vi "Тест_буфера_без_вырезания.vi"() -> ()   [LabVIEW 2017]
panel:
  out "2-х массив на выходе 2":dbl[][](array[numeric])
  out "Кол-во строк массив":i32
  in  "Размер окна":i32=4
  out "Выход последовательного массива":dbl[](array[numeric])
  in  "Последовательный массив":i32=16
  out "Array":dbl[][](array[numeric])
  in  "Размер окна буффера":i32
  out "Количество бит":i32
  in  "Количество бит":i32=8
  out "Биты на выходе":dbl[](array[numeric])
  # "3"
  # "15"
  # "7"
  # "3"
  # "7"
  # "15"
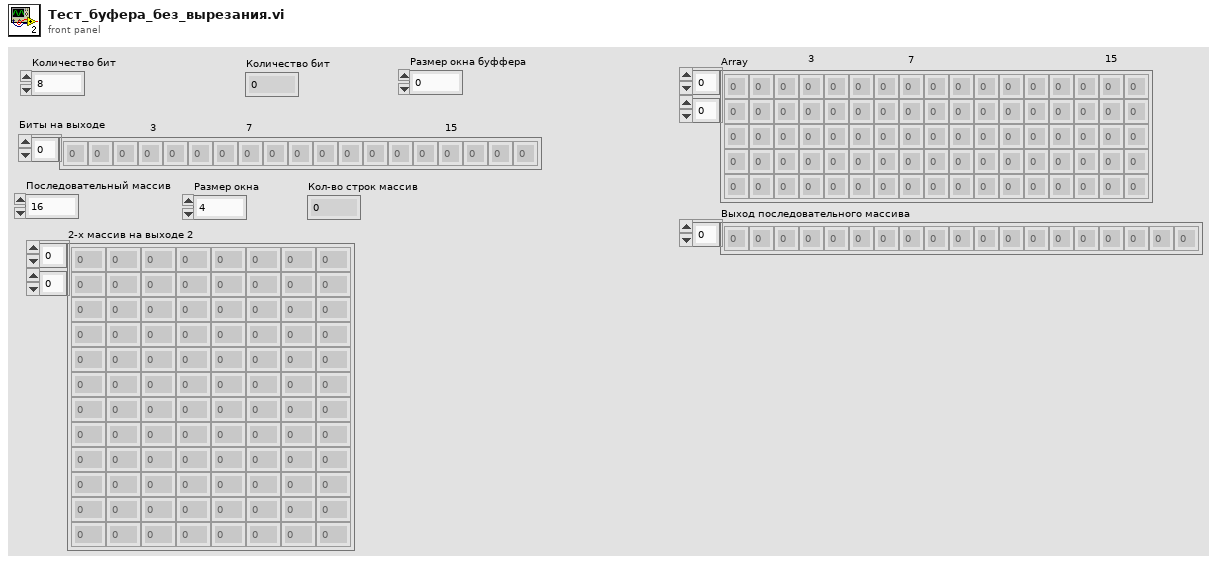
[diagram p1: front panel]
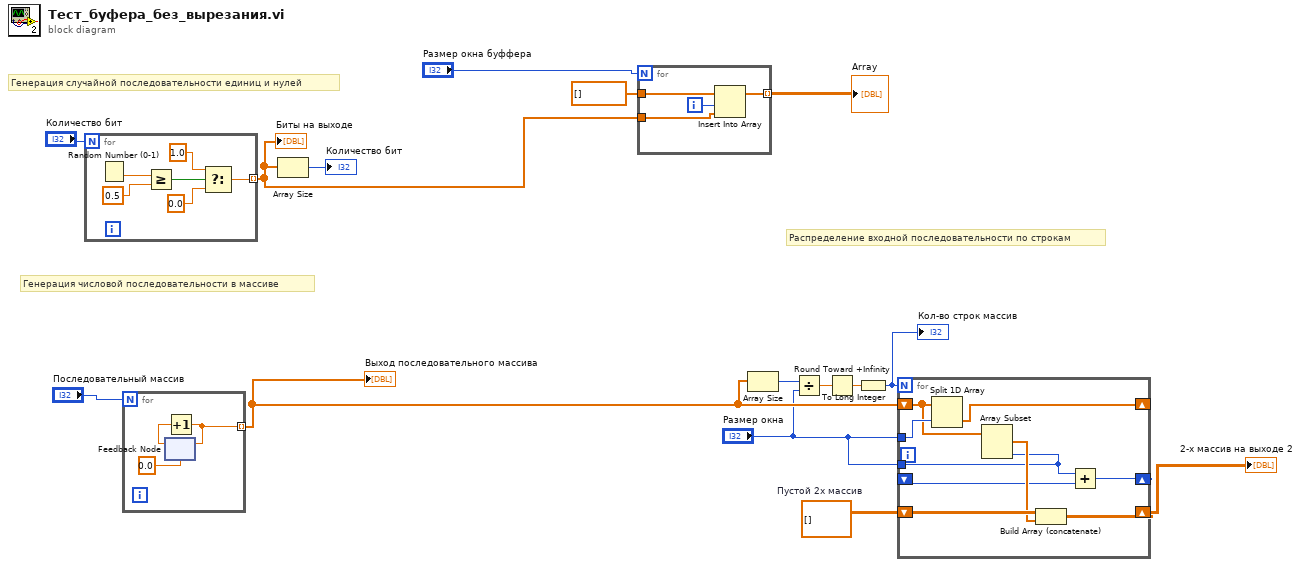
[diagram p0: block diagram]
diagram:
  w3 = dbl[][] []  # Пустой 2х массив
  # "Распределение входной последовательности по строкам"
  # "Генерация числовой последовательности в массиве"
  # "Генерация случайной последовательности единиц и нулей"
  n1 = for {
    N: "Количество бит" -> [_]
    tunnel: [w16] -> w10 mode=indexing
    n2 = Random Number (0-1)() -> (number: 0 to 1=w21:dbl)
    n3 = Greater Or Equal?(x=w21, y=0.5) -> (x >= y?=w19:bool)
    n4 = Select(t=1.0, s=w19, f=0.0) -> (s? t:f=w16:dbl)
  }
  "Биты на выходе" <- w10
  n5 = for {
    N: "Последовательный массив" -> [_]
    tunnel: [w22] -> w7 mode=indexing
    n6 = feedback #1(0.0) -> (w24:dbl)
    n7 = Increment(x=w24) -> (x+1=w22:dbl)
    n8 = feedback-in #1(w22) -> ()
  }
  "Выход последовательного массива" <- w7
  n9 = Array Size(array=w10) -> (size(s)=→"Количество бит":i32)
  n10 = for {
    N: "Размер окна буффера" -> [_]
    tunnel: w10 -> [w26]
    tunnel: dbl[] [] -> [w27]
    tunnel: [w28] -> w13 mode=indexing
    i -> [w25]
    n11 = Insert Into Array(array=w27, index=w25, new element=w26) -> (w28:dbl[])
  }
  "Array" <- w13
  n12 = Array Size(array=w7) -> (size(s)=w8:i32)
  n13 = Divide(x=w8, y="Размер окна") -> (x/y=w6:dbl)
  n14 = Round Toward +Infinity(x=w6) -> (ceil(x): smallest int >= x=w4:dbl)
  n15 = To Long Integer(number=w4) -> (32bit integer=w5:i32)
  "Кол-во строк массив" <- w5
  n16 = for {
    N: w5 -> [_]
    shift-right: [w37] -> _
    shift-left: w7 -> [w35]
    tunnel: "Размер окна" -> [w36]
    shift-right: [w32] -> w2
    shift-left: w3 -> [w34]
    shift-right: [w30] -> _
    shift-left: _ -> [w29]
    tunnel: "Размер окна" -> [w31]
    n17 = Split 1D Array(array=w35, index=w36) -> (second subarray=w37:dbl[])  [unwired: 1 out]
    n18 = Array Subset(array=w35, length=w31) -> (w33:dbl[])  [unwired: 1 in]
    n19 = Build Array (concatenate)(w34, w33) -> (w32:dbl[][])
    n20 = Add(x=w31, y=w29) -> (x+y=w30:i32)
  }
  "2-х массив на выходе 2" <- w2
